vi "CANopen Application.vi"() -> ()   [LabVIEW 2016]
doc: "This example demonstrates how to send and receive PDO messages triggered by a SYNC frame."
uses:
  <vilib>/userdefined/High Color/nirio_resource_hc.ctl
  <vilib>/Platform/TimedLoop/XDataNode/timing_clust.ctl
  <vilib>/Platform/TimedLoop/XDataNode/nitl_modes.ctl
  <vilib>/Platform/TimedLoop/XDataNode/wakeup.ctl
  <vilib>/FPGAPlugInAG/cRIO-9033/niLvFpga_Open_cRIO-9033.vi
  <vilib>/rvi/interface/common/dynamic/niFpgaDynamicAddResources.vi
  <vilib>/CANopenLib/CANOPEN.llb/CANopen Interface Create.vi
  <vilib>/CANopenLib/CANOPEN.llb/CANopen SDO Create.vi
  <vilib>/CANopenLib/CANOPEN.llb/CANopen SDO Close.vi
  <vilib>/CANopenLib/CANOPEN.llb/CANopen SYNC Create.vi
  <vilib>/CANopenLib/CANOPEN.llb/CANopen RPDO Create.vi
  <vilib>/CANopenLib/CANOPEN.llb/CANopen TPDO Create.vi
  <vilib>/CANopenLib/CANOPEN.llb/CANopen SYNC Start.vi
  <vilib>/CANopenLib/CANOPEN.llb/CANopen RPDO Start.vi
  <vilib>/CANopenLib/CANOPEN.llb/CANopen TPDO Start.vi
  <vilib>/CANopenLib/CANOPEN.llb/CANopen Convert To Data [U16].vi
  <vilib>/CANopenLib/CANOPEN.llb/CANopen Fetch from Data [I16].vi
  <vilib>/CANopenLib/CANOPEN.llb/CANopen SYNC Close.vi
  <vilib>/CANopenLib/CANOPEN.llb/CANopen RPDO Close.vi
  <vilib>/CANopenLib/CANOPEN.llb/CANopen TPDO Close.vi
  <vilib>/CANopenLib/CANOPEN.llb/CANopen Interface Close.vi
  <vilib>/FPGAPlugInAG/Dynamic/niLvFpga_Close_Dynamic.vi
  <vilib>/rvi/interface/nirviOpenFPGA/nirviOpenFPGA.xnode
  FPGA Bitfiles/project_FPGATarget_MainFPGA_S9ZLErdeBuw.lvbitx
  FPGA/MainFPGA.vi
  <vilib>/Platform/TimedLoop/XDataNode/XDataNode.xnode
  <vilib>/rvi/interface/nirviCloseFPGA/nirviCloseFPGA.xnode
  <vilib>/Platform/TimedLoop/XDataNode/XDNodeRunTimeDep.lvlib
panel:
  in  "error in":errorcluster
  in  "buffer size (0)":u16=10
  in  "PDO channel read":u8(ring) items=["PDO 1", "PDO 2", "PDO 3", "PDO 4"]
  in  "PDO channel write":u8(ring) items=["PDO 1", "PDO 2", "PDO 3", "PDO 4"]
  out "completion code":u32 format="%.0x"
  in  "batch SDO name":string="BatchSDO"
  in  "period (ms)":i64=10
  in  "stop":bool
  out "timestamp":timestamp=timestamp(11705972400 s since 1904-01-01)
  out "channel data read":dbl(knob) scale=0.0..10.0
  in  "channel data write":dbl(knob) scale=0.0..10.0
  out "CANopen raw data write":u8[](array[numeric])
  out "CANopen raw data read":u8[](array[numeric])
  in  "node-ID":u8=1 min=1 max=127 step=1
  in  "baud rate":u32(ring)=2 items=["1 Mbit/s"=0, "800 kbit/s"=1, "500 kbit/s"=2, "250 kbit/s"=3, "125 kbit/s"=4, "50 kbit/s"=6, "20 kbit/s"=7, "10 kbit/s"=8]
  in  "CANopen interface":u32(ring) items=["CANopen01", "CANopen02", "CANopen03", "CANopen04", "CANopen05", "CANopen06", "CANopen07", "CANopen08", "CANopen09", "CANopen10", "CANopen11", "CANopen12", "CANopen13", "CANopen14", "CANopen15", "CANopen16", "CANopen17", "CANopen18", "CANopen19", "CANopen20", "CANopen21", "CANopen22", "CANopen23", "CANopen24", "CANopen25", "CANopen26", "CANopen27", "CANopen28", "CANopen29", "CANopen30", "CANopen31", "CANopen32"]
  # "Overview: This example demonstrates how to send and receive PDO messages triggered by a SYNC frame. \nRequirements: Connect a CANopen module with a slave device.\nInstructions:\n1. Right-click BatchSDO in the NI CANopen for cRIO project and select Deploy from the shortcut menu.\n2. Specify the values of CANopen interface, baud rate of the CANopen interface and node-ID of the slave device.\n3. Specify the values of batch SDO name, PDO channel write and PDO channel read.\n4. Run this VI.\n5. Click STOP to stop the VI."
  # "Create CANopen interface and SYNC object"
  # "Configure and execute Batch SDO commands"
  # "Write RPDO messages"
  # "Read TPDO messages"
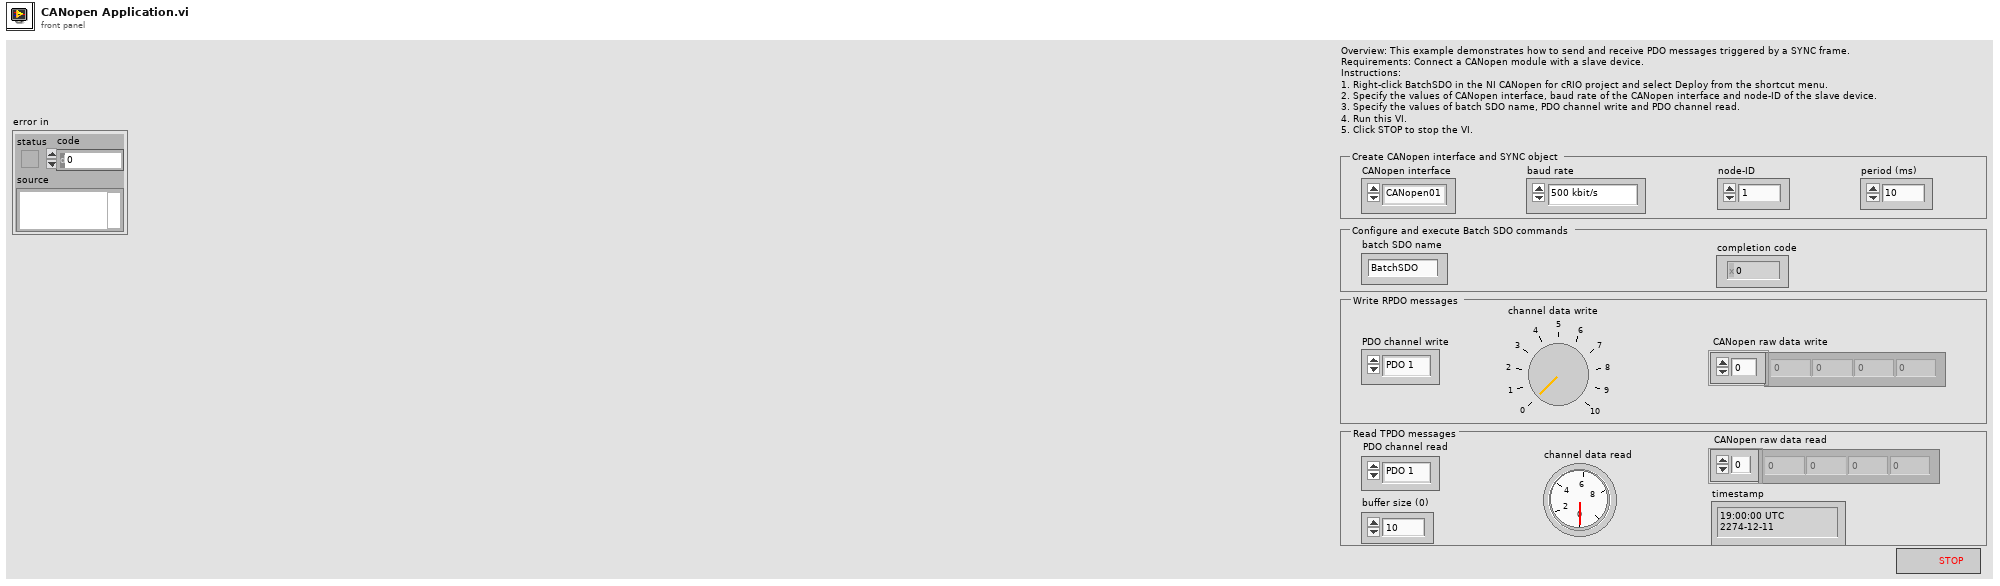
[diagram p1: front panel]
types:
  T1 = typedef "nirio_resource_hc.ctl" = tag
  T2 = typedef "XDNodeRunTimeDep.lvlib/timing_clust.ctl" = cluster{"Expected End [f-1]":u64, "Actual End [f-1]":u64, "Finished Late? [f-1]":bool, "Expected End [i-1]":u64, "Actual End [i-1]":u64, "Finished Late? [i-1]":bool, "Expected Start [i]":u64, "Actual Start [i]":u64, "Expected Start [f]":u64, "Actual Start [f]":u64, "Source Name":string, "Structure Name":string, "Period":i64, "Deadline":i64, "Offset":i64, "Start":i64, "Priority":i32, "Timeout":i32, "Mode":T3, "Wakeup Reason":T4, "Error":errorcluster, "Source Type":string, "Secondary Source Type":string, "Global End Time":u64, "Global Start Time":u64, "Frame Duration":u64, "Iteration Duration":u64, "Assigned CPU":i32, "I/O Scan Engine Mode":u32}
  T3 = typedef "XDNodeRunTimeDep.lvlib/nitl_modes.ctl" = enum32{"No Change", "Process missed periods, maintain original phase", "Discard missed periods, maintain original phase", "Process missed periods, ignore original phase", "Discard missed periods, ignore original phase"}
  T4 = typedef "XDNodeRunTimeDep.lvlib/wakeup.ctl" = enum32{"Normal", "Aborted", "Asynchronous wakeup", "Timing source error", "Timed loop error", "Timeout"}
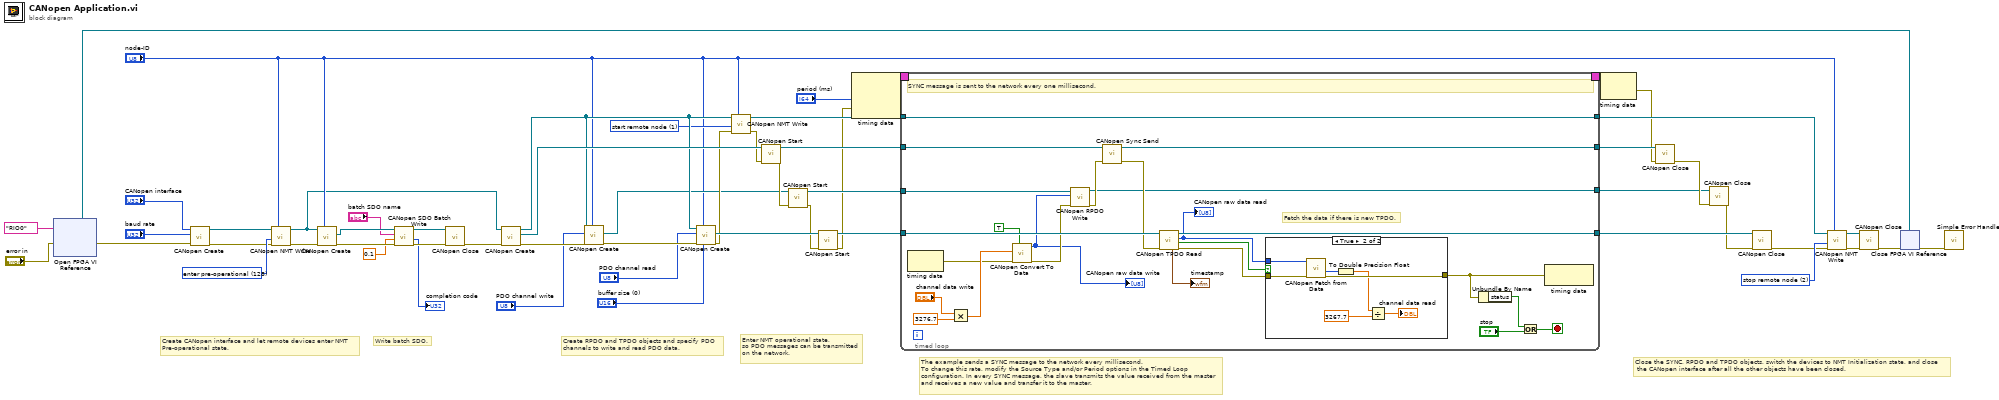
[diagram p0: block diagram]
diagram:
  w22 = u16 1 items=["start remote node"=1, "stop remote node"=2, "enter pre-operational"=128, "reset node"=129, "reset communication"=130] ("command")
  w45 = u16 2 items=["start remote node"=1, "stop remote node"=2, "enter pre-operational"=128, "reset node"=129, "reset communication"=130] ("command")
  w51 = u16 128 items=["start remote node"=1, "stop remote node"=2, "enter pre-operational"=128, "reset node"=129, "reset communication"=130] ("command")
  # "Close the SYNC, RPDO and TPDO objects, switch the devices to NMT Initialization state, and close\n the CANopen interface after all the other objects have been closed."
  # "The example sends a SYNC message to the network every millisecond.\nTo change this rate, modify the Source Type and/or Period options in the Timed Loop\nconfiguration. In every SYNC message, the slave transmits the value received from the master\nand receives a new value and transfer it to the master."
  # "Enter NMT operational state,\nso PDO messages can be transmitted\non the network."
  # "Create RPDO and TPDO objects and specify PDO \nchannels to write and read PDO data."
  # "Write batch SDO."
  # "Create CANopen interface and let remote devices enter NMT\nPre-operational state."
  n1 = xnode ("Open FPGA VI Reference")("error in"="error in", "resource name"=T1 "RIO0") -> ("FPGA VI Reference Out"=w1:refnum<k20>, "error out"=w4:errorcluster)
  n2 = call-poly <vilib>:"CANopen Create.vi"("error in (no error)"=w4, "baud rate"="baud rate", "interface name"="CANopen interface") -> ("error out"=w50:errorcluster, "interface object out"=w49:refnum<k20>)  [unwired: 7 in]
  n3 = call <vilib>:"CANopen NMT Write.vi"("node-ID (0)"="node-ID", "error in (no error)"=w50, "command"=w51, "interface object in"=w49) -> ("error out"=w38:errorcluster, "interface object out"=w7:refnum<k20>)  [unwired: 6 in]
  n4 = call-poly <vilib>:"CANopen Create.vi"("node-ID"="node-ID", "error in (no error)"=w38, "interface object in"=w7) -> ("error out"=w41:errorcluster, "SDO object out"=w42:refnum<k20>)  [unwired: 6 in, 1 out]
  n5 = call <vilib>:"CANopen SDO Batch Write.vi"("error in (no error)"=w41, "timeout (1s)"=0.1 ("timeout (0s)"), "batch SDO name"="batch SDO name", "SDO object in"=w42) -> ("error out"=w40:errorcluster, "completion code"=→"completion code":u32, "SDO object out"=w36:refnum<k20>)  [unwired: 5 in]
  n6 = call-poly <vilib>:"CANopen Close.vi"("error in (no error)"=w40, "SDO object in"=w36) -> ("error out"=w37:errorcluster)  [unwired: 9 in]
  n7 = call-poly <vilib>:"CANopen Create.vi"("error in (no error)"=w37, "interface object in"=w7) -> ("error out"=w26:errorcluster, "SYNC object out"=w25:refnum<k20>, "interface object out"=w24:refnum<k20>)  [unwired: 7 in]
  n8 = call-poly <vilib>:"CANopen Create.vi"("node-ID"="node-ID", "error in (no error)"=w26, "PDO channel"="PDO channel write", "interface object in"=w24) -> ("error out"=w16:errorcluster, "RPDO object out"=w15:refnum<k20>)  [unwired: 5 in, 1 out]
  n9 = call-poly <vilib>:"CANopen Create.vi"("buffer size (0)"="buffer size (0)", "node-ID"="node-ID", "error in (no error)"=w16, "PDO channel"="PDO channel read", "interface object in"=w24) -> ("error out"=w21:errorcluster, "TPDO object out"=w35:refnum<k20>)  [unwired: 4 in, 1 out]
  n10 = call <vilib>:"CANopen NMT Write.vi"("node-ID (0)"="node-ID", "error in (no error)"=w21, "command"=w22, "interface object in"=w24) -> ("error out"=w20:errorcluster, "interface object out"=w23:refnum<k20>)  [unwired: 6 in]
  n11 = call-poly <vilib>:"CANopen Start.vi"("error in (no error)"=w20, "SYNC object in"=w25) -> ("error out"=w19:errorcluster, "SYNC object out"=w48:refnum<k20>)  [unwired: 8 in]
  n12 = call-poly <vilib>:"CANopen Start.vi"("error in (no error)"=w19, "RPDO object in"=w15) -> ("error out"=w18:errorcluster, "RPDO object out"=w33:refnum<k20>)  [unwired: 8 in]
  n13 = call-poly <vilib>:"CANopen Start.vi"("error in (no error)"=w18, "TPDO object in"=w35) -> ("error out"=w14:errorcluster, "TPDO object out"=w32:refnum<k20>)  [unwired: 8 in]
  n14 = node-c288("period (ms)", w14) -> (w55:T2)  [unwired: 1 in]
  n15 = timed-loop {
    timing: w55 -> [_]
    timing-out: [_] -> w54
    tunnel: w48 -> [w79]
    tunnel: [w64] -> w17
    tunnel: [w78] -> w44
    tunnel: w23 -> [w78]
    tunnel: w33 -> [w71]
    tunnel: w32 -> [w72]
    tunnel: [w68] -> w29
    tunnel: [w67] -> w30
    stop <- w77 stop-if-true
    # "Fetch the data if there is new TPDO."
    # "SYNC message is sent to the network every one millisecond."
    n16 = node-c288() -> (w59:errorcluster)  [unwired: 1 in]
    n17 = Multiply(x="channel data write", y=3276.7) -> (x*y=w60:dbl)
    n18 = call-poly <vilib>:"CANopen Convert To Data.vi"("trim"=TRUE, "error in (no error)"=w59, "unsigned 16-bit integer"=w60) -> ("error out"=w66:errorcluster, "CANopen data out"=w56:u8[])  [unwired: 7 in]
    "CANopen raw data write" <- w56
    n19 = call <vilib>:"CANopen RPDO Write.vi"("error in (no error)"=w66, "data"=w56, "RPDO object in"=w71) -> ("error out"=w70:errorcluster, "RPDO object out"=w67:refnum<k20>)  [unwired: 7 in]
    n20 = call <vilib>:"CANopen Sync Send.vi"("error in (no error)"=w70, "SYNC object in"=w79) -> ("error out"=w69:errorcluster, "SYNC object out"=w64:refnum<k20>)  [unwired: 8 in]
    n21 = call <vilib>:"CANopen TPDO Read.vi"("error in (no error)"=w69, "TPDO object in"=w72) -> ("error out"=w73:errorcluster, "new data?"=w63:bool, "data"=w57:u8[], "TPDO object out"=w68:refnum<k20>, "timestamp"=→"timestamp":timestamp)  [unwired: 5 in]
    "CANopen raw data read" <- w57
    n22 = case shown="True" w63 {
      tunnel: w73 -> [w85 w92]
      tunnel: w57 -> [_ w91]
      tunnel: [w85 w90] -> w58
      frame False {
      }
      frame True {
        n23 = call-poly <vilib>:"CANopen Fetch from Data.vi"("error in (no error)"=w92, "CANopen data in"=w91) -> ("error out"=w90:errorcluster, "signed 16-bit integer"=w89:i16)  [unwired: 7 in, 1 out]
        n24 = To Double Precision Float(number=w89) -> (double precision float=w86:dbl)
        n25 = Divide(x=w86, y=3267.7) -> (x/y=→"channel data read":dbl)
      }
    }
    n26 = Unbundle By Name(w58) -> ("status"=w75:bool)
    n27 = Or(x=w75, y="stop") -> (x .or. y?=w77:bool)
    n28 = node-c288(w58) -> ()  [unwired: 1 out]
  }
  n29 = node-c288(w54) -> (w8:errorcluster)
  n30 = call-poly <vilib>:"CANopen Close.vi"("error in (no error)"=w8, "SYNC object in"=w17) -> ("error out"=w31:errorcluster)  [unwired: 9 in]
  n31 = call-poly <vilib>:"CANopen Close.vi"("error in (no error)"=w31, "RPDO object in"=w30) -> ("error out"=w28:errorcluster)  [unwired: 9 in]
  n32 = call-poly <vilib>:"CANopen Close.vi"("error in (no error)"=w28, "TPDO object in"=w29) -> ("error out"=w27:errorcluster)  [unwired: 9 in]
  n33 = call <vilib>:"CANopen NMT Write.vi"("node-ID (0)"="node-ID", "error in (no error)"=w27, "command"=w45, "interface object in"=w44) -> ("error out"=w47:errorcluster, "interface object out"=w46:refnum<k20>)  [unwired: 6 in]
  n34 = call-poly <vilib>:"CANopen Close.vi"("error in (no error)"=w47, "interface object in"=w46) -> ("error out"=w3:errorcluster)  [unwired: 9 in]
  n35 = xnode "Close FPGA VI Reference"("FPGA VI Reference In"=w1, "error in"=w3) -> ("error out"=w2:errorcluster)
  n36 = call <vilib>:"Simple Error Handler.vi"("error in (no error)"=w2) -> ()  [unwired: 4 in, 5 out]
